vi "socket_char_data.vi"() -> ()   [LabVIEW 2020]
panel:
  out "float output 3":dbl
  in  "index of float 3":i32
  out "float output 2":dbl
  in  "index of float 2":i32
  out "float output":dbl
  in  "index of float":i32
  out "data out":string
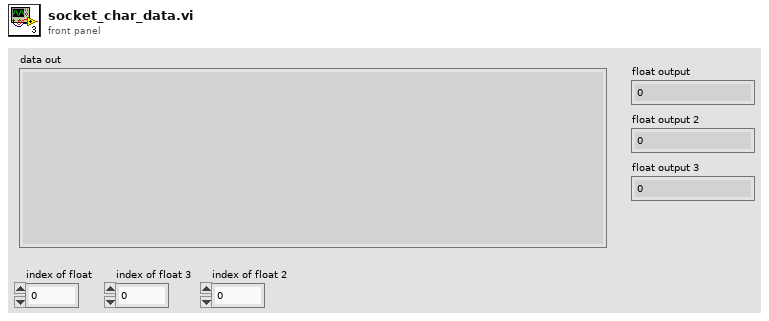
[diagram p1: front panel]
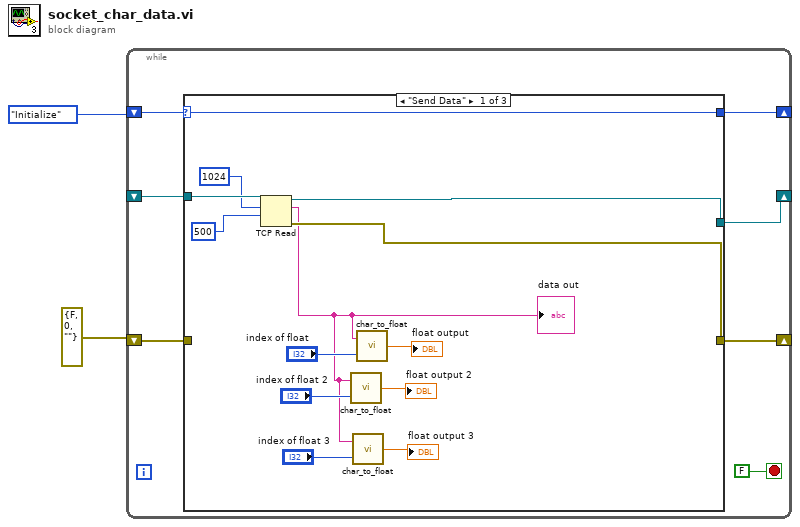
[diagram p0: block diagram]
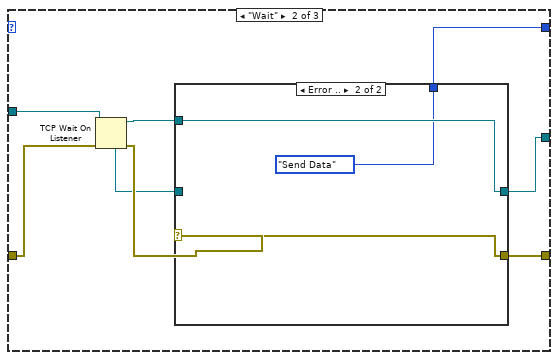
[diagram p2: hidden frame]
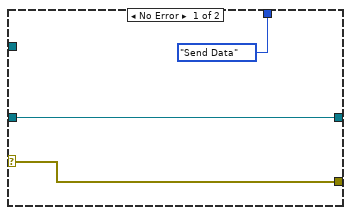
[diagram p3: hidden frame]
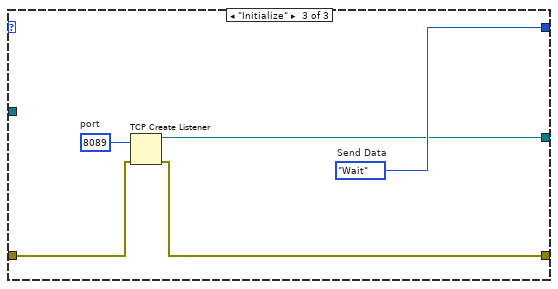
[diagram p4: hidden frame]
diagram:
  n1 = while {
    shift-right: [w8] -> _
    shift-left: enum16{"Initialize", "Send Data", "Wait"}."Initialize" -> [w9]
    shift-right: [w7] -> _
    shift-left: _ -> [w6]
    shift-right: [w3] -> _
    shift-left: errorcluster {"status"=FALSE, "code"=0, "source"=""} ("error in (no error)") -> [w4]
    stop <- FALSE stop-if-true
    n2 = case shown="\"Send Data\"" w9 {
      selector: w9 -> [w18 _ _]
      tunnel: [w18 w27 w40] -> w8
      tunnel: [w19 w25 w39] -> w7
      tunnel: w6 -> [w22 w30 _]
      tunnel: w4 -> [_ w29 w38]
      tunnel: [w17 w23 w37] -> w3
      frame "Send Data" {
        n3 = TCP Read(connection ID=w22, bytes to read=1024, 9:500 ("timeout ms (25000)")) -> (connection ID out=w19:refnum<k5>, data out=w10:string, error out=w17:errorcluster)  [unwired: 1 in, 1 out]
        "data out" <- w10
        n4 = call "char_to_float.vi"("index of float"="index of float 2", "data input"=w10) -> ("float output"=→"float output 2":dbl)
        n5 = call "char_to_float.vi"("index of float"="index of float 3", "data input"=w10) -> ("float output"=→"float output 3":dbl)
        n6 = call "char_to_float.vi"("index of float"="index of float", "data input"=w10) -> ("float output"=→"float output":dbl)
      }
      frame "Wait" {
        n7 = TCP Wait On Listener(8:w29, 11:w30) -> (0:w28:errorcluster, 3:w24:refnum<k5>, 4:w26:refnum<k5>)  [unwired: 4 out]
        n8 = case shown="Error .." w28 {
          selector: w28 -> [w31 w34]
          tunnel: [enum16{"Initialize", "Send Data", "Wait"}."Send Data" enum16{"Initialize", "Send Data", "Wait"}."Send Data"] -> w27
          tunnel: w26 -> [w32 _]
          tunnel: [w32 w36] -> w25
          tunnel: w24 -> [_ w36]
          tunnel: [w31 w34] -> w23
          frame No Error {
          }
          frame Error {
          }
        }
      }
      frame "Initialize" {
        w40 = enum16{"Initialize", "Send Data", "Wait"}."Wait"  # Send Data
        w41 = u16 8089  # port
        n9 = TCP Create Listener(8:w38, 10:w41) -> (0:w37:errorcluster, 3:w39:refnum<k5>)  [unwired: 4 out]
      }
    }
  }
